vi "Configuration Dialogue Box.vi"(8 "error in":errorcluster, 11 "Configuration Settings In":T1) -> (0 "error out":errorcluster, 3 "Configuration Settings Out":T1)   [LabVIEW 2021]
doc: "Shows the user the current settings and allows the user to change the settings of the DAQ inputs."
uses:
  controls/Configuration Settings.ctl
panel:
  in  "Cancel":bool
  in  "Ok":bool
  in  "Maximum Value":dbl
  in  "Minimum Value":dbl
  in  "Desired Sample Rate (Hz)":dbl
  in  "Number of Samples":i32
  in  "Physical Channels":tag
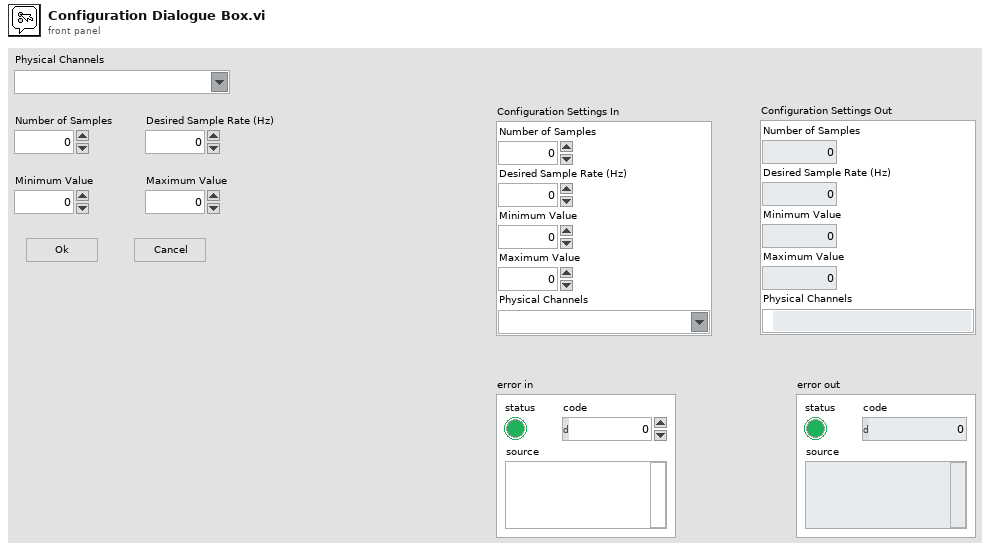
[diagram p1: front panel]
types:
  T1 = typedef "Configuration Settings.ctl" = cluster{"Number of Samples":i32, "Desired Sample Rate (Hz)":dbl, "Minimum Value":dbl, "Maximum Value":dbl, "Physical Channels":tag}
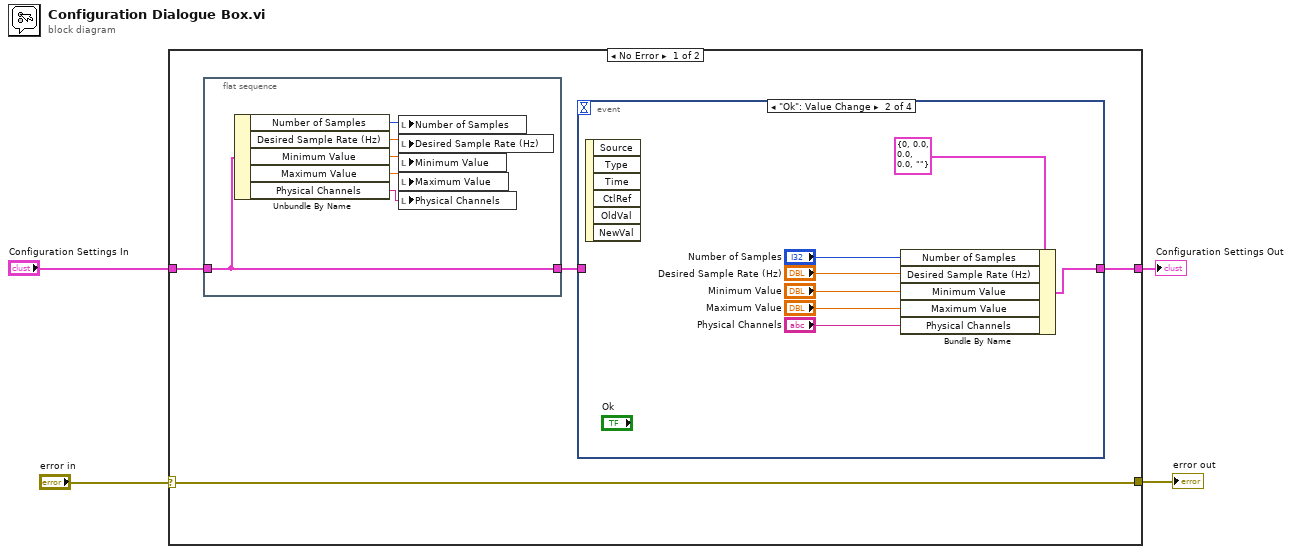
[diagram p0: block diagram]
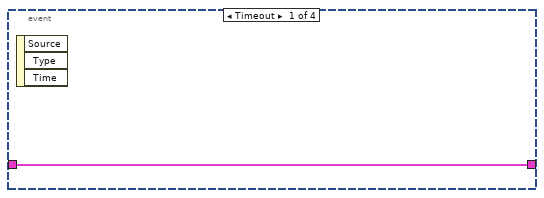
[diagram p2: hidden frame]
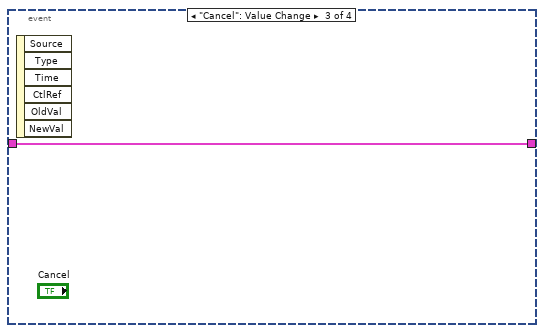
[diagram p3: hidden frame]
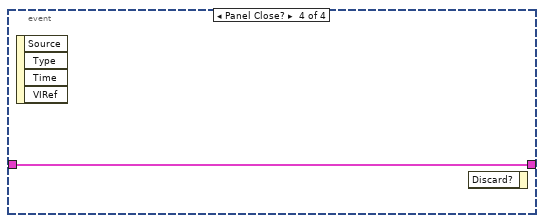
[diagram p4: hidden frame]
diagram:
  n1 = case shown="No Error" "error in" {
    selector: "error in" -> [w8 w26]
    tunnel: [w8 w26] -> w4
    tunnel: "Configuration Settings In" -> [w7 w25]
    tunnel: [w6 w25] -> w1
    frame No Error {
      n2 = flat-sequence {
        tunnel: w7 -> [w19]
        tunnel: [w19] -> _
        tunnel: [w19] -> w5
        frame #0 {
          n3 = Unbundle By Name(w19) -> ("Number of Samples"=w24:i32, "Desired Sample Rate (Hz)"=w23:dbl, "Minimum Value"=w22:dbl, "Maximum Value"=w21:dbl, "Physical Channels"=w20:tag)
          n4 = local write "Number of Samples"(w24) -> ()
          n5 = local write "Desired Sample Rate (Hz)"(w23) -> ()
          n6 = local write "Minimum Value"(w22) -> ()
          n7 = local write "Maximum Value"(w21) -> ()
          n8 = local write "Physical Channels"(w20) -> ()
        }
      }
      n9 = event shown="[1] \"Ok\": Value Change" {
        selector: _ -> [_ _ _ _]
        dyn-events: _ -> [_ _ _ _]
        timeout: _ -> [_ _ _ _]
        tunnel: [w9 w15 w17 w18] -> w6
        tunnel: w5 -> [w9 _ w17 w18]
        event Timeout {
          n10 = event-data() -> ()  [unwired: 1 in, 3 out]
        }
        event "Ok": Value Change {
          n11 = event-data() -> ()  [unwired: 1 in, 6 out]
          n12 = Bundle By Name(cluster=T1 {"Number of Samples"=0, "Desired Sample Rate (Hz)"=0.0, "Minimum Value"=0.0, "Maximum Value"=0.0, "Physical Channels"=""} ("Configuration Settings In"), "Number of Samples"="Number of Samples", "Desired Sample Rate (Hz)"="Desired Sample Rate (Hz)", "Minimum Value"="Minimum Value", "Maximum Value"="Maximum Value", "Physical Channels"="Physical Channels") -> (w15:T1)
        }
        event "Cancel": Value Change {
          n13 = event-data() -> ()  [unwired: 1 in, 6 out]
        }
        event Panel Close? {
          n14 = event-data() -> ()  [unwired: 1 in, 4 out]
          n15 = event-data() -> ()  [unwired: 2 in, 1 out]
        }
      }
    }
    frame Error {
    }
  }
  "Configuration Settings Out" <- w1
  "error out" <- w4
